vi "Get Parameter.vi"(8 "error in (no error)":errorcluster, 11 "Stepper3D in":refnum<class "Stepper3D.lvclass">) -> (0 "error out":errorcluster, 2 "Parameter":refnum<class "AbstractData.lvclass">, 3 "Stepper3D out":refnum<class "Stepper3D.lvclass">)   [LabVIEW 2014, in "Stepper3D.lvclass"]
uses:
  Stepper3D.lvclass
  Framework/Model/Data/AbstractData/AbstractData.lvclass
  Framework/Model/Data/DataSingleElement/DataSingleElement.lvclass
  Framework/Interfaces/Observable Actor/Observable Actor.lvclass
  wlmData.dll
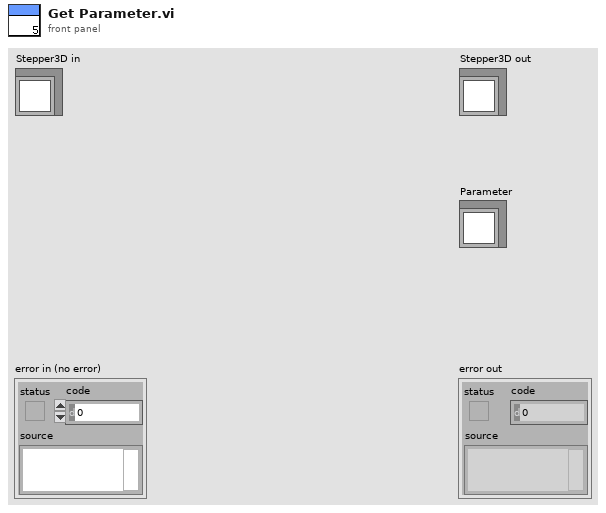
[diagram p1: front panel]
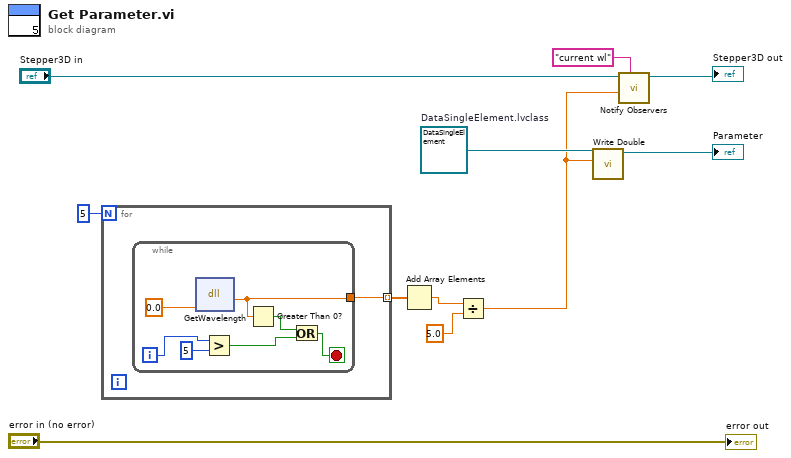
[diagram p0: block diagram]
diagram:
  w6 = refnum<class "DataSingleElement.lvclass"> refnum  # DataSingleElement.lvclass
  n1 = for {
    N: 5 -> [_]
    tunnel: [w12] -> w4 mode=indexing
    n2 = while {
      tunnel: [w13] -> w12
      i -> [w18]
      stop <- w15 stop-if-true
      n3 = dll-call lib="wlmData.dll" fn="GetWavelength"("arg1"=0.0) -> ("return type"=w13:dbl)  [unwired: 4 in, 2 out]
      n4 = Greater?(x=w18, y=5) -> (0:w14:bool)
      n5 = Greater Than 0?(x=w13) -> (x > 0?=w16:bool)
      n6 = Or(x=w16, y=w14) -> (x .or. y?=w15:bool)
    }
  }
  n7 = Add Array Elements(numeric array=w4) -> (sum=w3:dbl)
  n8 = Divide(x=w3, y=5.0) -> (x/y=w1:dbl)
  n9 = call "Write Double.vi"("value"=w1, "DataSingleElement in"=w6) -> ("DataSingleElement out"=→"Parameter":refnum<class "DataSingleElement.lvclass">)  [unwired: 8 in, 1 out]
  n10 = call "Notify Observers.vi"("name"="current wl", "value"=w1, "Observable Actor in"="Stepper3D in") -> ("Observable Actor out"=→"Stepper3D out":refnum<class "Stepper3D.lvclass">)  [unwired: 7 in, 1 out]
  "error out" <- "error in (no error)"
